vi "LF2R IDE Regist Command.vi"(8 "error in (no error)":errorcluster, 11 "LF2R IDE in":refnum<class "Main Panel.lvclass">) -> (0 "error out":errorcluster, 3 "LF2R IDE out":refnum<class "Main Panel.lvclass">, 5 "Event Registration Refnum":refnum<event-registration>)   [LabVIEW 2018, in "Main Panel.lvlib" / "Main Panel.lvclass"]
uses:
  Main Panel.lvclass
  LF2R IDE Cmd Data.ctl
  LF2R IDE Cmd.ctl
  Main Panel.lvclass/Main Panel.ctl
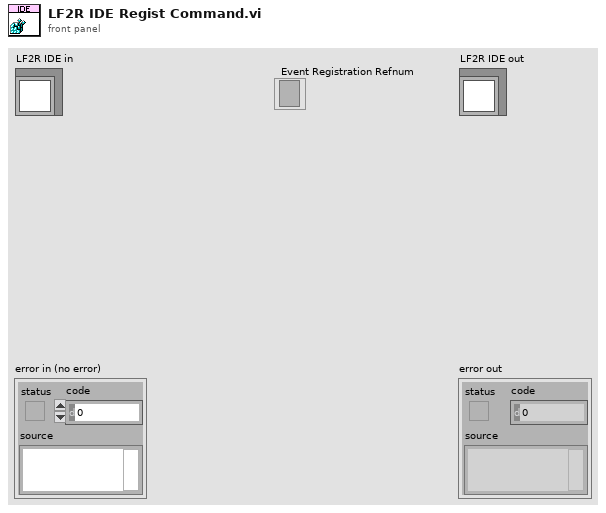
[diagram p1: front panel]
types:
  T1 = typedef "Main Panel.lvlib/Main Panel.lvclass/LF2R IDE Cmd Data.ctl" = cluster{"Command":T2, "Data":variant}
  T2 = typedef "Main Panel.lvlib/Main Panel.lvclass/LF2R IDE Cmd.ctl" = enum16{"Save Data File", "Write Configuration", "Save Configuration", "Update Frame Image"}
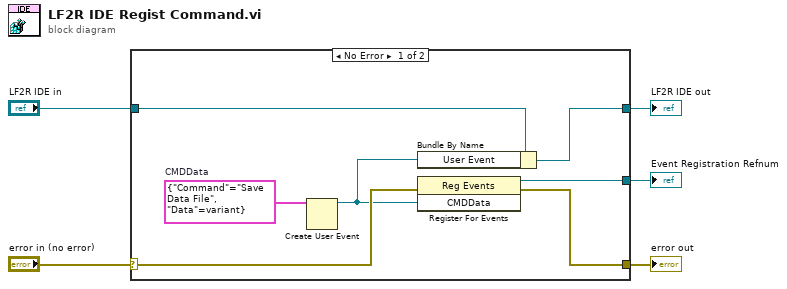
[diagram p0: block diagram]
diagram:
  n1 = case shown="No Error" "error in (no error)" {
    selector: "error in (no error)" -> [w9 w14]
    tunnel: [w8 w14] -> w4
    tunnel: [w7 w13] -> w2
    tunnel: "LF2R IDE in" -> [w12 w13]
    tunnel: [w10 _] -> w1
    frame No Error {
      w11 = T1 {"Command"=enum."Save Data File", "Data"=variant}  # CMDData
      n2 = Create User Event(user event datatype=w11) -> (user event=w6:refnum<user-event>)  [unwired: 1 in, 1 out]
      n3 = Bundle By Name(cluster=w12, "User Event"=w6) -> (w7:refnum<class "Main Panel.lvclass">)
      n4 = register-events(error in=w9, w6) -> (reference out=w10:refnum<event-registration>, error out=w8:errorcluster)  [unwired: 1 in]
    }
    frame Error {
    }
  }
  "error out" <- w4
  "LF2R IDE out" <- w2
  "Event Registration Refnum" <- w1
